vi "Logging queue size check.vi"(11 "Queues refs":T1) -> (2 "Elements in logging queue":i32, 3 "Registered peak value of remaining elements":i32)   [LabVIEW 2020]
uses:
  User Interface/Queue/Message Queue/Typedefs/All Message Queues.ctl
  User Interface/Queue/Message Queue/Typedefs/Message Cluster.ctl
  Typedefs/Logging queue element.ctl
  Typedefs/Imaging Protocols enum.ctl
  Typedefs/Frame Size.ctl
  Typedefs/Acquired points count.ctl
  Typedefs/Read Write Enum.ctl
  Global Variables/General Globals.vi
panel:
  # "Background priority"
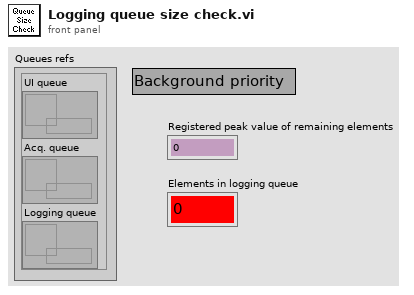
[diagram p1: front panel]
types:
  T1 = typedef "All Message Queues.ctl" = cluster{"UI queue":refnum<queue>, "Acq. queue":refnum<queue>, "Logging queue":refnum<queue>}
  T2 = typedef "Read Write Enum.ctl" = enum16{"Read", "Write"}
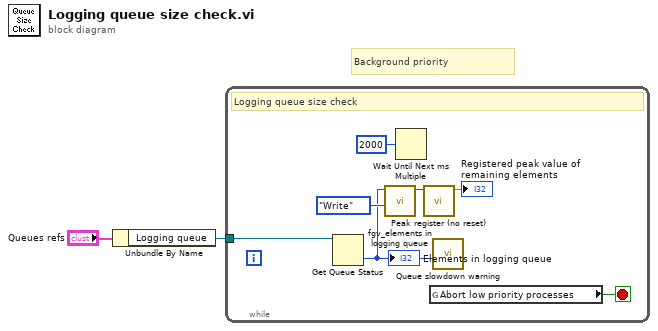
[diagram p0: block diagram]
diagram:
  # "Background priority"
  n1 = Unbundle By Name("Queues refs") -> ("Logging queue"=w2:refnum<queue>)
  n2 = while {
    tunnel: w2 -> [w7]
    stop <- w3 stop-if-true
    # "Logging queue size check"
    n3 = Get Queue Status(queue=w7) -> (# elements in queue=w5:i32)  [unwired: 2 in, 7 out]
    "Elements in logging queue" <- w5
    n4 = call "fgv_elements in logging queue.vi"("Function"=Read_Write_Enum."Write", "Elements in logging queue"=w5) -> ("Elements in logging queue"=w9:i32)  [unwired: 8 in, 1 out]
    n5 = Wait Until Next ms Multiple(millisecond multiple=u32 2000) -> ()  [unwired: 1 out]
    n6 = call <userlib>:"Peak register (no reset).vi"("Value in"=w9) -> ("Registered peak value"=→"Registered peak value of remaining elements":dbl)  [unwired: 10 in]
    n7 = global read "General Globals.vi" "Abort low priority processes"() -> (w3:bool)
    n8 = call "Queue slowdown warning.vi"("# elements in queue in"=w5) -> ()  [unwired: 11 in]
  }
